vi "Get Accelerometer Angle.vi"() -> (0 "Accelerometer Angle":dbl)   [LabVIEW 2012]
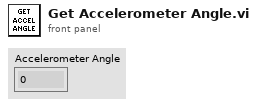
[diagram p1: front panel]
types:
  T1 = typedef "WPI_AccelerometerDevRef.ctl" = cluster{"DevStatus":errorcluster, "Analog Module":T2, "Analog Channel":T3, "Scaling":T4}
  T2 = typedef "FPGA_TypedefAnalogModule.ctl" = enum16{"Analog Module 1", "Analog Module 2"}
  T3 = typedef "FPGA_AIChannel.ctl" = enum8{"AI 1", "AI 2", "AI 3", "AI 4", "AI 5", "AI 6", "AI 7", "AI 8", "Invalid"}
  T4 = typedef "WPI_AccelerometerScaling.ctl" = cluster{"Gain (VoltsPerG)":dbl, "Center Voltage":dbl}
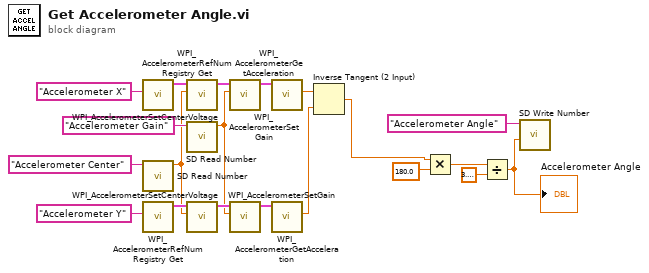
[diagram p0: block diagram]
diagram:
  n1 = call <vilib>:"WPI_AccelerometerRefNum Registry Get.vi"("refnum name"="Accelerometer X") -> ("AccelerometerDevRef"=w8:T1)  [unwired: 9 in, 1 out]
  n2 = call <vilib>:"SD Read Number.vi"("Name"="Accelerometer Center" ("refnum name")) -> ("Numeric"=w3:dbl)  [unwired: 8 in, 2 out]
  n3 = call <vilib>:"WPI_AccelerometerRefNum Registry Get.vi"("refnum name"="Accelerometer Y") -> ("AccelerometerDevRef"=w7:T1)  [unwired: 9 in, 1 out]
  n4 = call <vilib>:"WPI_AccelerometerSetCenterVoltage.vi"("Center Voltage"=w3, "AccelerometerDevRef"=w8) -> ("AccelerometerDevRef"=w18:T1)  [unwired: 1 in, 8 out]
  n5 = call <vilib>:"SD Read Number.vi"("Name"="Accelerometer Gain" ("refnum name")) -> ("Numeric"=w4:dbl)  [unwired: 8 in, 2 out]
  n6 = call <vilib>:"WPI_AccelerometerSetCenterVoltage.vi"("Center Voltage"=w3, "AccelerometerDevRef"=w7) -> ("AccelerometerDevRef"=w19:T1)  [unwired: 1 in, 8 out]
  n7 = call <vilib>:"WPI_AccelerometerSetGain.vi"("Gain (VoltsPerG)"=w4, "AccelerometerDevRef"=w18) -> ("AccelerometerDevRef"=w17:T1)  [unwired: 1 in, 8 out]
  n8 = call <vilib>:"WPI_AccelerometerSetGain.vi"("Gain (VoltsPerG)"=w4, "AccelerometerDevRef"=w19) -> ("AccelerometerDevRef"=w20:T1)  [unwired: 1 in, 8 out]
  n9 = call <vilib>:"WPI_AccelerometerGetAcceleration.vi"("AccelerometerDevRef"=w17) -> ("Acceleration"=w12:dbl)  [unwired: 1 in, 9 out]
  n10 = call <vilib>:"WPI_AccelerometerGetAcceleration.vi"("AccelerometerDevRef"=w20) -> ("Acceleration"=w11:dbl)  [unwired: 1 in, 9 out]
  n11 = Inverse Tangent (2 Input)(1:w11, 2:w12) -> (0:w13:dbl)
  n12 = Multiply(x=w13, y=180.0) -> (x*y=w15:dbl)
  n13 = Divide(x=w15, y=3.141592653589793) -> (x/y=w2:dbl)
  "Accelerometer Angle" <- w2
  n14 = call <vilib>:"SD Write Number.vi"("Numeric"=w2, "Name"="Accelerometer Angle") -> ()  [unwired: 8 in, 2 out]
